vi "Write value.vi"(8 "error in (no error)":errorcluster, 10 "value":cluster{"t0":dbl, "dt":dbl, "y":dbl[]}, 11 "UserDefinedWaveform in":refnum<class "UserDefinedWaveform.lvclass">) -> (0 "error out":errorcluster, 3 "UserDefinedWaveform out":refnum<class "UserDefinedWaveform.lvclass">)   [LabVIEW 2014, in "UserDefinedWaveform.lvclass"]
uses:
  UserDefinedWaveform.lvclass
  UserDefinedWaveform.lvclass/UserDefinedWaveform.ctl
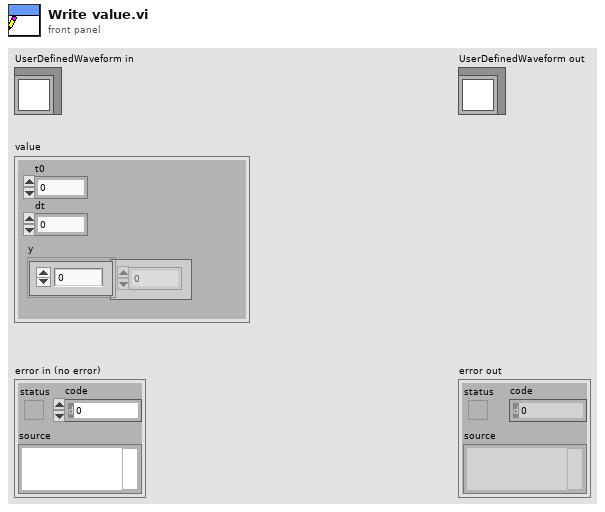
[diagram p1: front panel]
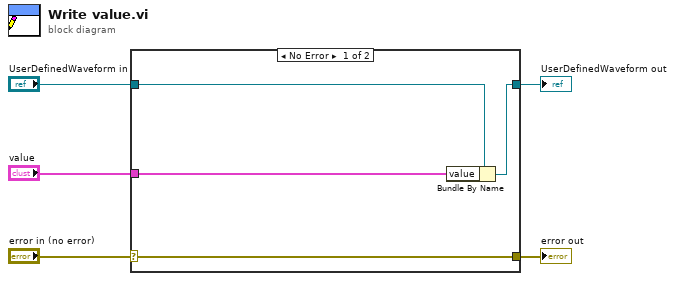
[diagram p0: block diagram]
diagram:
  n1 = case shown="No Error" "error in (no error)" {
    selector: "error in (no error)" -> [w9 w10]
    tunnel: [w9 w10] -> w4
    tunnel: [w7 w11] -> w2
    tunnel: "UserDefinedWaveform in" -> [w8 w11]
    tunnel: "value" -> [w6 _]
    frame No Error {
      n2 = Bundle By Name(cluster=w8, "value"=w6) -> (w7:refnum<class "UserDefinedWaveform.lvclass">)
    }
    frame Error {
    }
  }
  "error out" <- w4
  "UserDefinedWaveform out" <- w2
